vi "RT Main AB Oct 24 2019.vi"() -> ()   [LabVIEW 2018]
uses:
  Type Defs/BL Measurement States.ctl
  <vilib>/Platform/TimedLoop/XDataNode/timing_clust.ctl
  <vilib>/Platform/TimedLoop/XDataNode/nitl_modes.ctl
  <vilib>/Platform/TimedLoop/XDataNode/wakeup.ctl
  <vilib>/FPGAPlugInAG/myRIO-1900/niLvFpga_Open_myRIO-1900.vi
  <vilib>/rvi/interface/common/dynamic/niFpgaDynamicAddResources.vi
  <vilib>/Utility/error.llb/Error Cluster From Error Code.vi
  <vilib>/rvi/errors/niLvFpgaAdjustHostInterfaceError.vi
  <vilib>/FPGAPlugInAG/Dynamic/niLvFpga_Close_Dynamic.vi
  <vilib>/Platform/TimedLoop/XDataNode/XDataNode.xnode
  <vilib>/rvi/interface/nirviOpenFPGA/nirviOpenFPGA.xnode
  UNCC Watt balance Oct19/FPGA Bitfiles/UNCCWattbalanceO_FPGATarget_fpganestedFORW&R_sb-Oe1PDHtY.lvbitx
  <vilib>/rvi/interface/nirviReadWriteControl/nirviReadWriteControl.xnode
  <vilib>/rvi/interface/nirviCloseFPGA/nirviCloseFPGA.xnode
  <vilib>/Platform/TimedLoop/XDataNode/XDNodeRunTimeDep.lvlib
  NiFpgaLv.dll
  <vilib>/rvi/interface/Simulation/niFpgaSimulationCallBeginRW.vi
panel:
  out "Velocity (m/s)":dbl
  out "BL":dbl=13.526543432913298
  out "Cycles 2":dbl=2.5
  out "Time period 2":dbl=0.039999999999999994 format="%.4f"
  out "Amplitude (EMF)":dbl=0.42519521147770484 format="%.6f"
  out "Cycles":dbl=2.5
  out "Time period":dbl=0.039999999999999994 format="%.4f"
  out "Amplitude (CP)":dbl=0.00020011592768339807 format="%.6f"
  in  "no. data points":u16=500
  in  "Measure":bool
  in  "Period (us)":i64=200
  in  "EMF Gain":dbl=1.0
  in  "offset (V)":dbl format="%#_13g"
  in  "frequency (Hz)":dbl=25.0 format="%#_13g"
  in  "amplitude (V)":dbl=0.9 format="%#_13g"
  out "Late? [i-1]":bool
  in  "Stop Button":bool
  out "?":cluster{dbl, dbl}(graph)
  out "sine fit debug":dbl[][](graph)=[[-8.368204220516664e-06, -1.4715763614446807e-05, -2.4183697758518094e-05, -3.0424447258800375e-05, -3.976268367487069e-05, -4.5911881837740506e-05, -5.50670155789859e-05, -6.107125745761935e-05, -7.000514213345132e-05, -7.588731556220149e-05, -8.456180478203151e-05, -9.026850481407448e-05, -9.866071074354942e-05, -0.00010419193737888519, -0.00011230186001800507, -0.000117596579031692, -0.00012534792559927975, -0.00013041376626943556, -0.00013782179532172663, -0.00014264349909211586, -0.00014962428856981548, -0.00015414845049361426, -0.00016074014678731094, -0.00016495913758640153, -0.00017110070647115364, -0.00017500689686741834, -0.0001806754505088728, -0.0001842612112241939, -0.00018941860323176213, -0.00019267630498802198, -0.0001972843889711155, -0.0002002292903245494, -0.00020430332483940364, -0.00020683624517448153, -0.00021252768665028907, -0.00021548784655995844, -0.0002172654683613836, -0.0002196458031341074, -0.0002210572195858827, -0.00022286535849977868, -0.00022388768176755108, -0.0002251083662663838, -0.00022572633779391788, -0.00022635956787768734, -0.0002266113340555716, -0.0002266342218899247, -0.00022649689488380602, -0.000225955216137449, -0.00022539827883485657, -0.00022429966278590712, -0.00022333074446495864, -0.00022165230327906364, -0.00022029429177411228, -0.00021799787906068323, -0.0002162812914841997, -0.00021338216579947197, -0.00021127648503898553, -0.00020782042205166543, -0.00020533327738529375, -0.00020134316492973427, -0.00019848981491371278, -0.0001939198773212078, -0.00019072320978988963, -0.00018563448128538072, -0.00018208686696064813, -0.00017650223537848844, -0.00017261130353845913, -0.00016654602743488406, -0.00016234992447014657, -0.00015583452095762693, -0.00015131798831194586, -0.00014437534522483478, -0.00013962230495750486, -0.00013227531013015545, -0.00012723235729435276, -0.00011949626928300042, -0.00011423206738178433, -0.00010617554968948836, -0.00010068246944474112, -9.23284099058547e-05, -8.667511482063566e-05, -7.802351343515875e-05, -7.219474495323252e-05, -6.331426522422447e-05, -5.732528190182644e-05, -4.822355310740498e-05, -4.210487205700597e-05, -3.2835299143994996e-05, -2.6579291087477307e-05, -1.715713261211225e-05, -1.0824831774417512e-05, -1.24245845858066e-06, 5.18139371652653e-06, 1.4801913422951904e-05, 2.1256282710529914e-05, 3.0968353754367744e-05, 3.7453240154416565e-05, 4.7172940476372095e-05, 5.360442192959699e-05, 6.322494163602237e-05, 6.958775958618793e-05, 7.907858156461232e-05, 8.534221889924771e-05, 9.464993820284721e-05, 0.00010079150708759933, 0.0001098932358820208, 0.00011589747776065425, 0.00012475506965530916, 0.0001305762088591177, 0.0001391972931321238, 0.00014483532966110742, 0.00015316650136564073, 0.00015862143521979945, 0.00016660928940903606, 0.00017182771564154593, 0.00017948751087172127, 0.0001844694294825823, 0.0001917553900849901, 0.00019647028396173148, 0.00020336715138013635, 0.00020780739124464037, 0.00021426938981033606, 0.00021841208782824963, 0.00022443158826311845, 0.00022826911515632384, 0.00023377745395730651, 0.00023729455116956825, 0.00024232224544913555, 0.00024550365442421826, 0.00025001255779178165, 0.00025285827852968544, 0.0002568331324290094, 0.00025930501853914573, 0.0002623414712299921, 0.0002623414712299921, 0.0002623414712299921, 0.0002623414712299921, 0.0002623414712299921, 0.0002623414712299921, 0.0002623414712299921, 0.0002623414712299921, 0.0002623414712299921, 0.0002623414712299921, 0.0002623414712299921, 0.0002623414712299921, 0.0002623414712299921, 0.0002623414712299921, 0.0002623414712299921, 0.0002623414712299921, 0.0002623414712299921, 0.0002623414712299921, 0.0002623414712299921, 0.0002623414712299921, 0.0002623414712299921, 0.0002623414712299921, 0.0002623414712299921, 0.0002623414712299921, 0.0002623414712299921, 0.0002609605718906876, 0.00025733666478477794, 0.00025471219311228765, 0.00025048557303507935, 0.00024752541312541, 0.00024281051924866863, 0.00023946889543311405, 0.00023426572775683957, 0.00023060367426034142, 0.00022488171567206302, 0.00022090686177273901, 0.00021472714649739834, 0.0002104394921952484, 0.00020380964951096321, 0.00019926259975281132, 0.00019220551749393465, 0.0001873609258891923, 0.00017993763828066584, 0.00017486416833239232, 0.00016706704609609834, 0.0001617494392480583, 0.0001536166287745853, 0.00014808540213924953, 0.00013964742054106837, 0.00013393309123090768, 0.0001251899385080183, 0.00011929250652303274, 0.00011032047545661226, 0.00010424757007491947, 9.506954849932095e-05, 8.890509178021571e-05, 7.955159680791e-05, 7.324218380456838e-05, 6.375136182614398e-05, 5.738854387597842e-05, 4.777565344767075e-05, 4.136705982879898e-05, 3.1731281566138194e-05, 2.528454155667789e-05, 1.5664021850252515e-05, 9.270686787616142e-06, -2.964279719853011e-07, -6.651616644033151e-06, -1.609666295375132e-05, -2.2360300288386722e-05, -3.169090742633932e-05, -3.783247631109144e-05, -4.700286860857226e-05, -5.303762759967652e-05, -6.201728794421471e-05, -6.792997848543571e-05, -7.666550193020736e-05, -8.240271907472114e-05, -9.091699345407936e-05, -9.645584936753283e-05, -0.00010466495262218286, -0.00011001307658269371, -0.00011787886232204706, -0.0001230515128858507, -0.00013056635183178965, -0.0001354490898271205, -0.00014262061125776276, -0.00014724395379709168, -0.00015398823565314246, -0.00015834455345835173, -0.00016463870790545793, -0.0001686669667516059, -0.00017452625234600297, -0.00017823408151120733, -0.00018360509330607133, -0.00018700775134656753, -0.0001918599722294276, -0.00019491168347650942, -0.00019923748416924783, -0.00020194587790103294, -0.00020572999984741437, -0.00020807981750766737, -0.00021127648503898553, -0.0002132295802371179, -0.00021589982757831447, -0.00021748671742679703, -0.00021958476890916577, -0.00022076730701740992, -0.00022227027480659772, -0.0002230866075651921, -0.00022404026732990518, -0.0002244446190701435, -0.00022481082441979332, -0.00022483371225414644, -0.0002246048339106153, -0.0002242691456734363, -0.00022343755435860651, -0.00022269751438118917, -0.0002212632100950607, -0.00022013407693364048, -0.0002181352060668019, -0.00021660935044326098, -0.00021402302516135917, -0.00021210044707569762, -0.0002089571844912034, -0.00020664551322153893, -0.00020293005477821683, -0.00020024454888078482, -0.00019598741169110575, -0.00019295858827837704, -0.000184749485023727, -0.00017945476601004007, -0.00017572404901048256, -0.00016991816836290944, -0.00016588228023864377, -0.00015958812579153756, -0.0001552623250987991, -0.00014853330179898374, -0.00014390232998153708, -0.0001367842134977188, -0.00013189384622427021, -0.00012435611944397817, -0.00011922924454888077, -0.00011137871736576284, -0.00010600770557089886, -9.782911942871964e-05, -9.227500495903076e-05, -8.381413552649647e-05, -7.809217693821809e-05, -6.937191204968184e-05, -6.349736789904938e-05, -5.456348322321741e-05, -4.852109495399546e-05, -3.938884904710317e-05, -3.3232021606115636e-05, -2.392430230251614e-05, -1.766829424599845e-05, -8.223247936280279e-06, -1.8985763767032463e-06, 7.668538382898196e-06, 1.404661488929916e-05, 2.3659505317606828e-05, 3.009861604894943e-05, 3.9742023589727915e-05, 4.6173505042952805e-05, 5.578639547126048e-05, 6.213395486519063e-05, 7.164003539985044e-05, 7.790367273448582e-05, 8.726479698490926e-05, 9.343688298213219e-05, 0.00010259201672337759, 0.00010864966354883496, 0.00011757591894654922, 0.0001234580923752994, 0.00013219361582007106, 0.00013789268657399633, 0.0001463459267284129, 0.00015187715336374867, 0.00016001759311533938, 0.000165319941407144, 0.00017312469292155572, 0.00017822867998230002, 0.0001856672261470619, 0.0001905423348642751, 0.0001975689000106809, 0.00020214646688130364, 0.00020879156812182424, 0.00021307922242397417, 0.00021925130842119712, 0.00022323379159863886, 0.00022897100874315265, 0.00023264069151776853, 0.0002378972641408669, 0.0002412236294001861, 0.00024597666966751596, 0.00024895208813342074, 0.0002531863374887467, 0.0002558184384393548, 0.00025951863832644143, 0.0002617997924836351, 0.0002623414712299921, 0.0002623414712299921, 0.0002623414712299921, 0.0002623414712299921, 0.0002623414712299921, 0.0002623414712299921, 0.0002623414712299921, 0.0002623414712299921, 0.0002623414712299921, 0.0002623414712299921, 0.0002623414712299921, 0.0002623414712299921, 0.0002623414712299921, 0.0002623414712299921, 0.0002623414712299921, 0.0002623414712299921, 0.0002623414712299921, 0.0002623414712299921, 0.0002623414712299921, 0.0002623414712299921, 0.0002623414712299921, 0.0002623414712299921, 0.0002623414712299921, 0.0002623414712299921, 0.0002596407067763247, 0.00025720696705677695, 0.0002532931473823946, 0.000250493202313197, 0.0002460605917268107, 0.00024288681202984567, 0.00023792778125333774, 0.00023444883043166446, 0.00022897100874315265, 0.0002251716282405358, 0.00021924367914307944, 0.00021512386895951898, 0.0002087305338968826, 0.00020432844042296712, 0.00019750786578573928, 0.00019282348902146873, 0.00018559856264400258, 0.00018067004897996545, 0.0001678528617422219, 0.0001599107832216915, 0.00015450925431435673, 0.00014624674611288274, 0.00014061633886201683, 0.00013206391809207009, 0.00012625803744449696, 0.00011743096266231285, 0.00011144960861803251, 0.00010237076765796416, 9.629023299815366e-05, 8.702828936326041e-05, 8.081042769733124e-05, 7.1418786334437e-05, 6.509411477485997e-05, 5.559566351831787e-05, 4.9217587011916905e-05, 3.962758441796235e-05, 3.322662007720827e-05, 2.3628988205136012e-05, 1.722802386438194e-05, 7.668538382898196e-06, 1.3057204327326442e-06, 0.0], [0.01724705128400751, 0.030827166333521522, 0.04379693913361917, 0.0648537467384836, 0.07721317728916488, 0.09750705708225885, 0.11047682988235649, 0.1304655385507423, 0.14343531135083995, 0.16296626333216346, 0.17547827944519884, 0.19485664586416826, 0.20706349085249548, 0.22598410058440263, 0.23742801776095937, 0.2560434563681584, 0.26870805804354786, 0.2861028121519141, 0.29724155820376263, 0.31387338450035845, 0.3254698872392693, 0.34133878572409465, 0.3523249462135892, 0.3678886735737063, 0.377501564002014, 0.3929127057997771, 0.40252559622808476, 0.41610571127759877, 0.4258711872682605, 0.43823061781894185, 0.4458598959366463, 0.45776156980026533, 0.46584860460503213, 0.4765295939698184, 0.48339594427575244, 0.4936191769534765, 0.5003329416970564, 0.5088777331888855, 0.5143708134336328, 0.5221526771136913, 0.5265776584219599, 0.533444008727894, 0.5364957199749758, 0.5421413857820772, 0.5448879259044508, 0.5485499794009489, 0.550533591711552, 0.5531275462715716, 0.5549585730198207, 0.5557215008315911, 0.5558740863939452, 0.5563318430810075, 0.5554163297068829, 0.5541956452080502, 0.5523646184598011, 0.5503810061491979, 0.5482448082762407, 0.5438198269679722, 0.5413784579703067, 0.5357327921632054, 0.5311552252925826, 0.5239837038619404, 0.5191009658666096, 0.5110139310618428, 0.5053682652547414, 0.4957553748264337, 0.48843126783343743, 0.4786657918427757, 0.47103651372507116, 0.4595925965485144, 0.4508952194943313, 0.43853578894365, 0.43029616857652914, 0.41641088240230695, 0.40740833422341566, 0.3926075346750689, 0.3829946442467612, 0.3671257457619359, 0.3576654408959823, 0.34149137128644874, 0.3314207241710788, 0.31417855562506664, 0.3030398095732181, 0.2857976410272059, 0.274048552725941, 0.25772189755405334, 0.2462779803774966, 0.22766254177029763, 0.2172867235302195, 0.19851869936066643, 0.18722736774646376, 0.1686119291392648, 0.1564050841509376, 0.13763705998138454, 0.12619314280482777, 0.10635701969879607, 0.09369241802340661, 0.07553473610326988, 0.06348047667729678, 0.04410211025832735, 0.03159009414529197, 0.012822069975738903, 0.000615224987411702, -0.01830538474449546, -0.030207058608114477, -0.04989059615179208, -0.06225002670247338, -0.08117063643438055, -0.09307231029799956, -0.1121455055922608, -0.12374200833117166, -0.14251003250072472, -0.1538013641149274, -0.17287455940918864, -0.18431847658574538, -0.2011028884446953, -0.21392007568243884, -0.23039931641668057, -0.2426061614050078, -0.25954315882631174, -0.27068190487816035, -0.28655080336298566, -0.2969266216030638, -0.3129481056502433, -0.3233239238903214, -0.3384298945633763, -0.3489582983658085, -0.3625384134153225, -0.37230388940598425, -0.38527366220608195, -0.39381845369791096, -0.40739856874742497, -0.41472267574042126, -0.42662434960404033, -0.4344062132840989, -0.4449346170865311, -0.45225872407952744, -0.46126127225841873, -0.46766986587729054, -0.4756043151197032, -0.4807922242397422, -0.48842150235744675, -0.492236141416299, -0.498949906159879, -0.502306788531669, -0.5073421120893539, -0.5096308955246652, -0.5131403634588093, -0.5151239757694125, -0.5174127592047238, -0.5181756870164943, -0.5197015426400352, -0.5195489570776811, -0.5192437859529729, -0.5184808581412025, -0.516039489143537, -0.5148188046447043, -0.5119196789599766, -0.5088679677128948, -0.5036800585928558, -0.5009335184704822, -0.4952878526633808, -0.49147321360452856, -0.4841491066115322, -0.4788086119291391, -0.4710267482490805, -0.4653810824419792, -0.45531043532660925, -0.44890184170773745, -0.43822085234295116, -0.4310493309123089, -0.41960541373575216, -0.41090803668156906, -0.3985486061308878, -0.3900038146390587, -0.37581335734012833, -0.36665822359888295, -0.35139966736347394, -0.3417867769351663, -0.3265282206997573, -0.3153894746479087, -0.2992154050383752, -0.2889921723606511, -0.271902589376993, -0.2604586722004363, -0.24306391809207006, -0.2313148297908051, -0.21254680562125203, -0.20018737507057074, -0.1826400353998504, -0.16982284816210683, -0.15074965286784558, -0.13747470894303976, -0.11794375696171625, -0.10558432641103493, -0.08513786105558688, -0.0727784305049056, -0.0527897218365198, -0.03920960678700579, -0.019220898118619996, -0.0060985397561682565, 0.014195340036925713, 0.027165112837023362, 0.04745899263011733, 0.060428765430214984, 0.08026488853624669, 0.09399758914811479, 0.11307078444237603, 0.12604055724247368, 0.14618185147321355, 0.1589990387109571, 0.17837740512992656, 0.19073683568060784, 0.20981003097486908, 0.22247463265025855, 0.24093748569510345, 0.25207623174695204, 0.2703864992294428, 0.2827459297801241, 0.2990725849520117, 0.31066908769092255, 0.32745349954987246, 0.338439660039367, 0.3540033873994841, 0.36453179120191637, 0.3794851763126172, 0.3895558234279871, 0.41320658559287105, 0.42678670064238505, 0.43502632100950595, 0.4476909226848954, 0.45562537192730806, 0.4666115324168026, 0.47317271159802843, 0.484311457649877, 0.49010970901933243, 0.4994174283229319, 0.5050630941300333, 0.5134553000595082, 0.5191009658666096, 0.5258147306101895, 0.5297819552313958, 0.5357327921632054, 0.5390896745349953, 0.5432094847185558, 0.5458034392785752, 0.5496180783374275, 0.5506861772739061, 0.5528223751468634, 0.5535853029586338, 0.5541956452080502, 0.5540430596456961, 0.5535853029586338, 0.5528223751468634, 0.5506861772739061, 0.5483973938385948, 0.5464137815279916, 0.5430568991562017, 0.538479332285579, 0.5348172787890808, 0.5290190274196254, 0.5239837038619404, 0.5174225246807146, 0.5117768588736132, 0.5030794818194301, 0.4975864015746828, 0.4873631688969588, 0.48171750308985745, 0.4699684147885925, 0.4617287944214717, 0.45028487724491495, 0.44189267131543997, 0.42861772739063414, 0.41992035033645103, 0.40588247859987475, 0.39626958817156704, 0.3811636174985122, 0.3713981415078504, 0.3562921708347955, 0.3451534247829469, 0.3286741840487052, 0.318145780246273, 0.3007510261379067, 0.28945969452370407, 0.27267528266475416, 0.26062102323878106, 0.24414178250453933, 0.23178235195385805, 0.2143875978454918, 0.2020281672948105, 0.18448082762409015, 0.17090071257457615, 0.15350595846620987, 0.14190945572729904, 0.12268367487068371, 0.11062941544471058, 0.09170880571280343, 0.0801123029738926, 0.060733936554923165, 0.04745899263011733, 0.028843554022918355, 0.016789294596945243, -0.0016735584478996465, -0.01479591681035139, -0.033411355417550366, -0.04546561484352348, -0.06484398126249291, -0.07674565512611192, -0.09597143598272728, -0.10802569540870038, -0.12572562064177484, -0.1368643666936234, -0.15517463417611418, -0.16783923585150368, -0.1856917466469322, -0.1975934205105512, -0.2148355890565634, -0.2268898484825365, -0.24321650365442415, -0.2549655919556891, -0.271750003814639, -0.2822784076170712, -0.29784213497718837, -0.3080653676549124, -0.32408685170209184, -0.3336997421303995, -0.3485005416787462, -0.3579608465446998, -0.37215130384363015, -0.38176419427193786, -0.39427621038497324, -0.40236324518974, -0.41487526130277536, -0.42280971054518807, -0.43379587103468253, -0.44142514915238706, -0.4508854540183406, -0.45775180432427465, -0.46736469475258235, -0.47285777499732956, -0.4844542777362404, -0.49147321360452856, -0.495593023788089, -0.5013912751575444, -0.503985229717564, -0.5082576254634784, -0.5106989944611439, -0.5135981201458716, -0.5146662190823502, -0.516039489143537, -0.5168024169553075, -0.5166498313929534, -0.5169550025176616, -0.5149713902070584, -0.5139032912705798, -0.5103938233364357, -0.5096308955246652, -0.5053584997787508, -0.502306788531669, -0.497271464973984, -0.49345682591513174, -0.48659047560919766, -0.48170773761386676, -0.47453621618322456, -0.46889055037612326, -0.4598880021972319, -0.45393716526542244, -0.44371393258769837, -0.43684758228176435, -0.4250984939804994, -0.41807955811221126, -0.40572012756153, -0.39702275050734687, -0.3840529777072492, -0.3747452584036497, -0.36024962998001114, -0.35124708180111985, -0.3364462822527731, -0.3259178784503409, -0.31004897996551556, -0.29952057616308336, -0.2833465065535498, -0.2715974182522849, -0.25527076308039726, -0.24306391809207006, -0.2253639928589956, -0.21376749012008475, -0.19545722263759396, -0.18370813433632902, -0.16524528129148414, -0.1521229229290324, -0.13320231319712525, -0.12084288264644394, -0.10131193066512043, -0.08834215786502278, -0.06804827807192879, -0.0558414330836016, -0.03570013885286172, -0.022730366052764066, -0.0030468285090864584]]
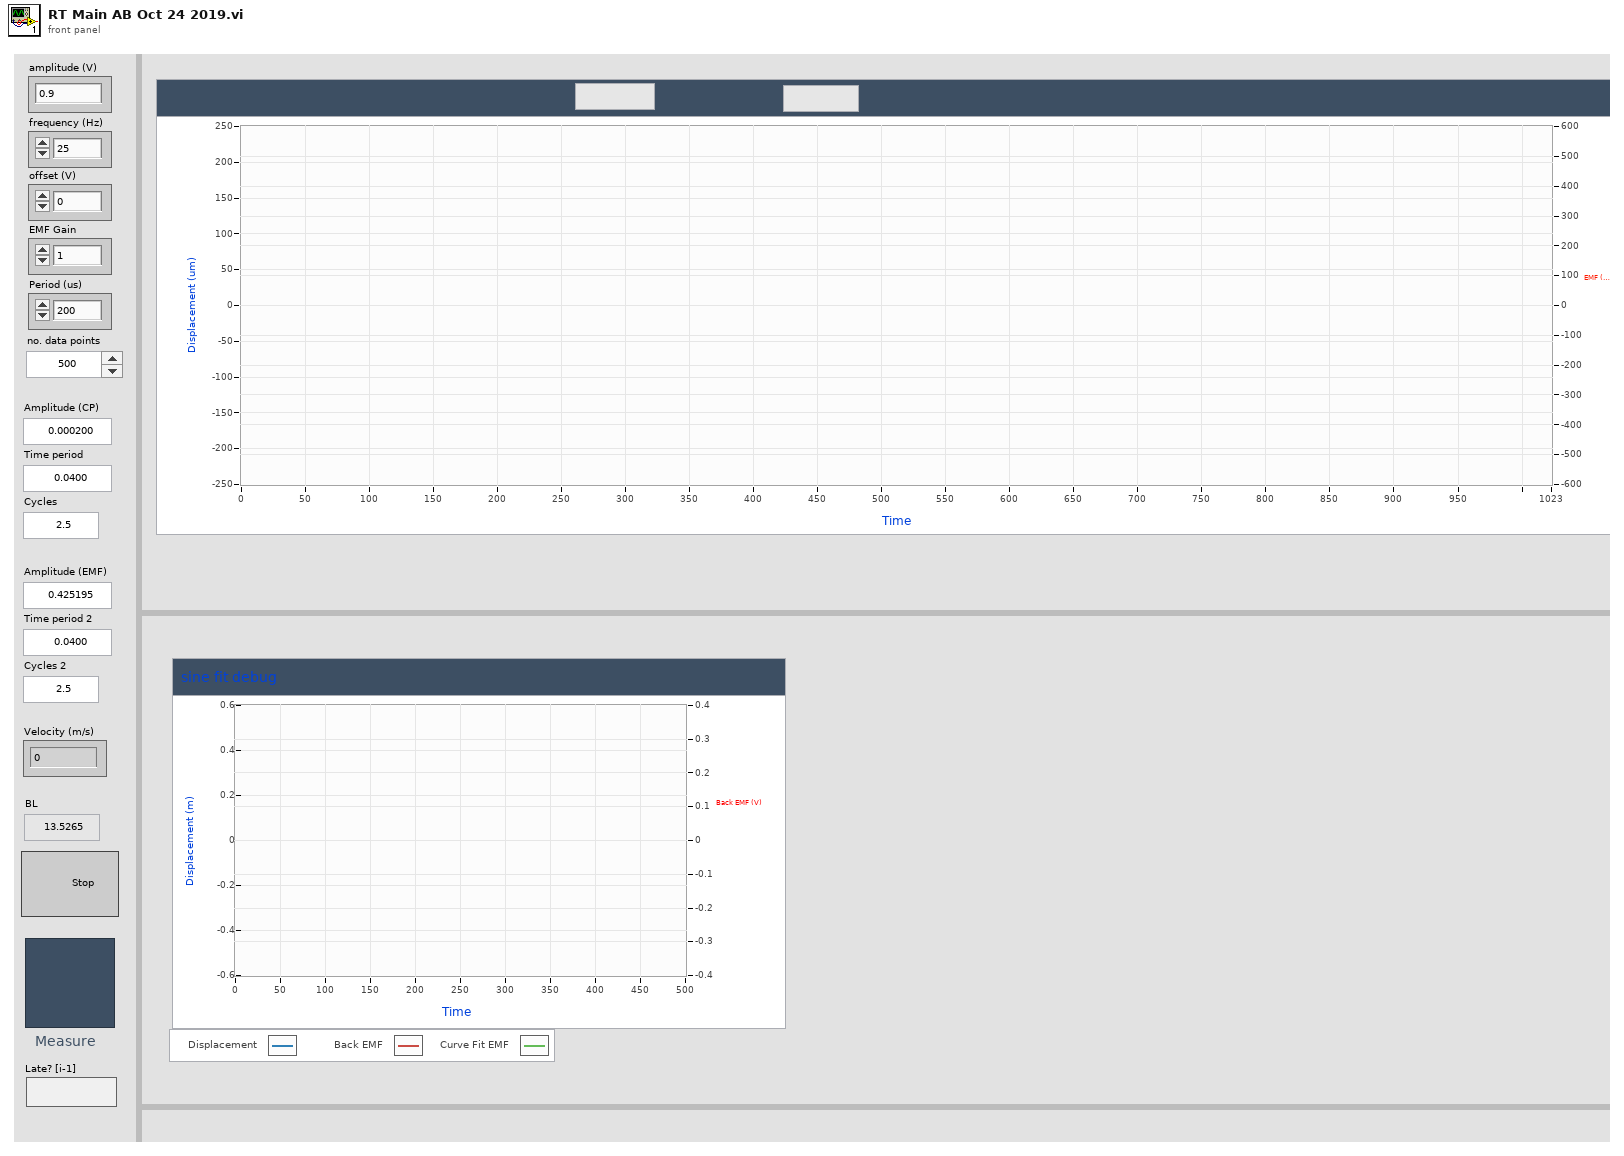
[diagram p1: front panel]
types:
  T1 = typedef "BL Measurement States.ctl" = enum16{"idle", "initialize", "collect data", "prepare data", "fit sine", "calculate BL", "exit meas"}
  T2 = typedef "XDNodeRunTimeDep.lvlib/timing_clust.ctl" = cluster{"Expected End [f-1]":u64, "Actual End [f-1]":u64, "Finished Late? [f-1]":bool, "Expected End [i-1]":u64, "Actual End [i-1]":u64, "Finished Late? [i-1]":bool, "Expected Start [i]":u64, "Actual Start [i]":u64, "Expected Start [f]":u64, "Actual Start [f]":u64, "Source Name":string, "Structure Name":string, "Period":i64, "Deadline":i64, "Offset":i64, "Start":i64, "Priority":i32, "Timeout":i32, "Mode":T3, "Wakeup Reason":T4, "Error":errorcluster, "Source Type":string, "Secondary Source Type":string, "Global End Time":u64, "Global Start Time":u64, "Frame Duration":u64, "Iteration Duration":u64, "Assigned CPU":i32, "I/O Scan Engine Mode":u32}
  T3 = typedef "XDNodeRunTimeDep.lvlib/nitl_modes.ctl" = enum32{"No Change", "Process missed periods, maintain original phase", "Discard missed periods, maintain original phase", "Process missed periods, ignore original phase", "Discard missed periods, ignore original phase"}
  T4 = typedef "XDNodeRunTimeDep.lvlib/wakeup.ctl" = enum32{"Normal", "Aborted", "Asynchronous wakeup", "Timing source error", "Timed loop error", "Timeout"}
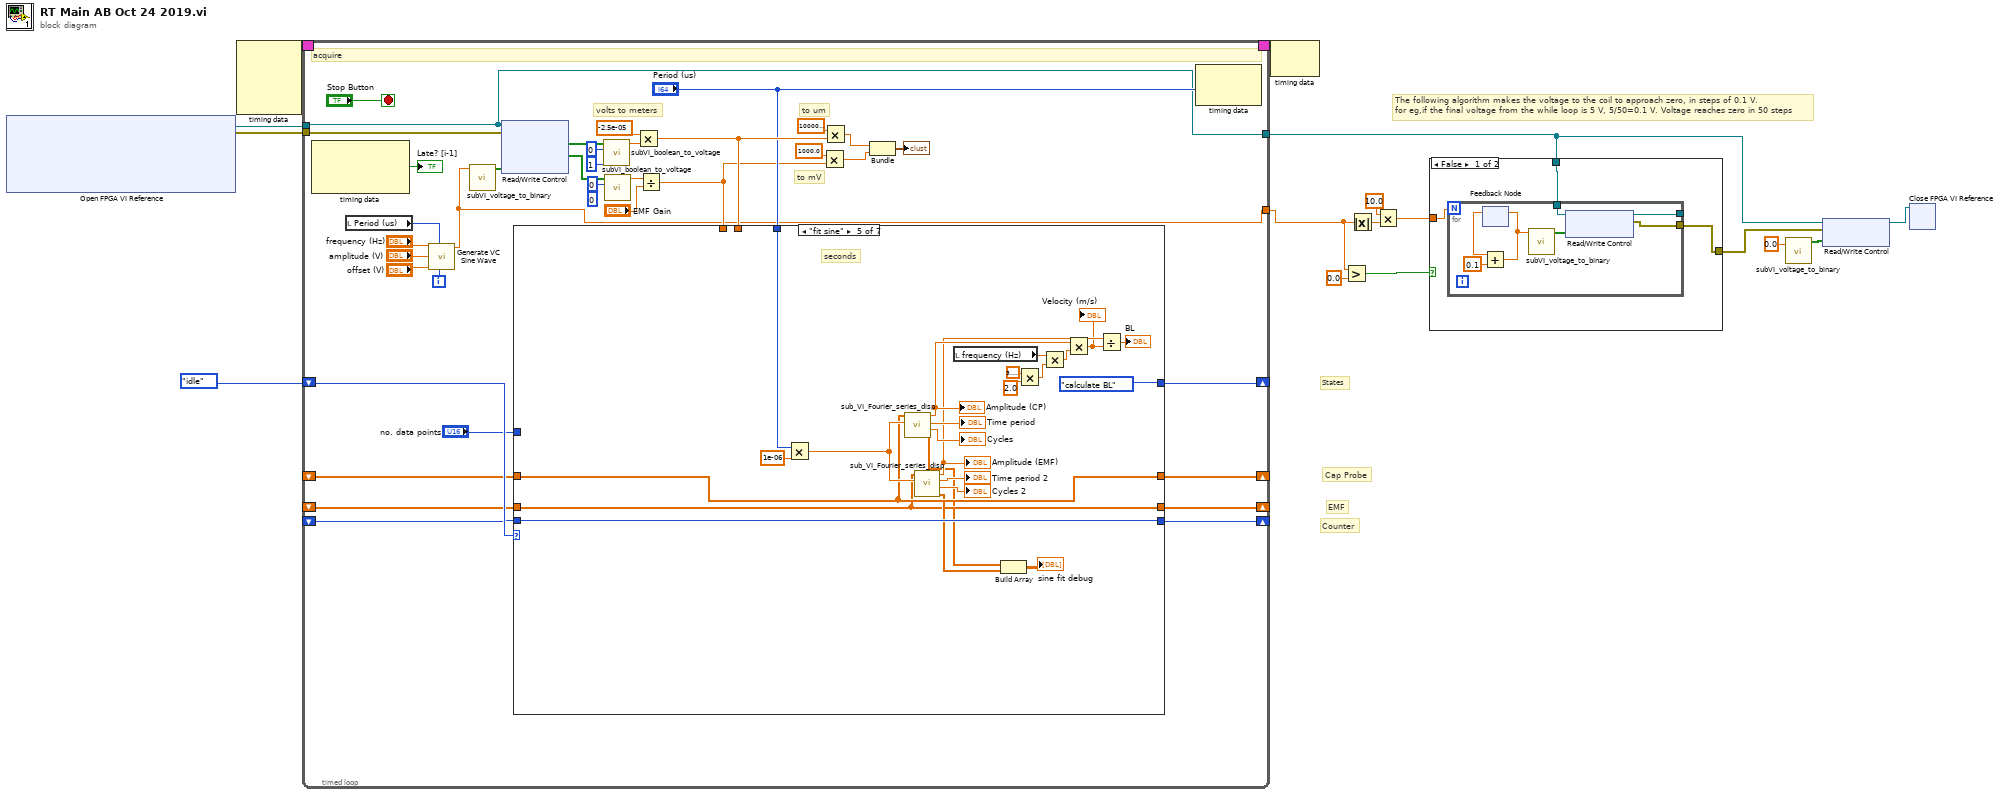
[diagram p0: block diagram]
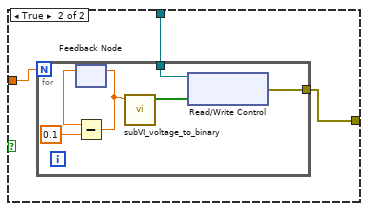
[diagram p2: hidden frame]
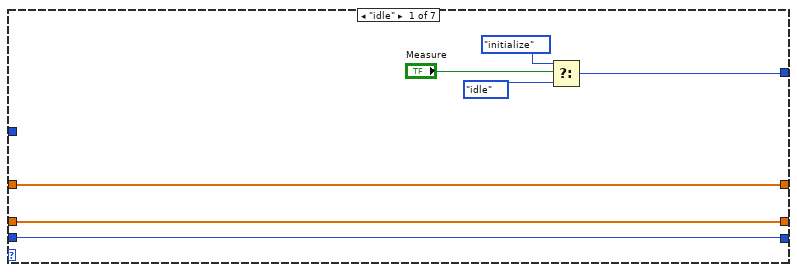
[diagram p3: hidden frame]
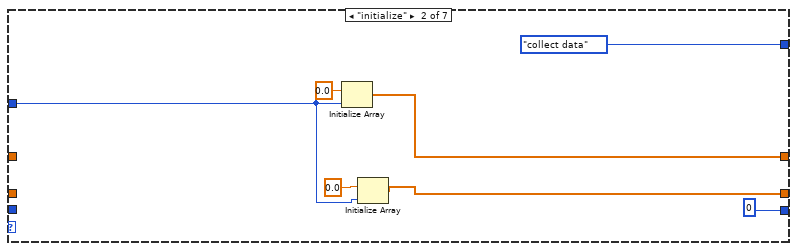
[diagram p4: hidden frame]
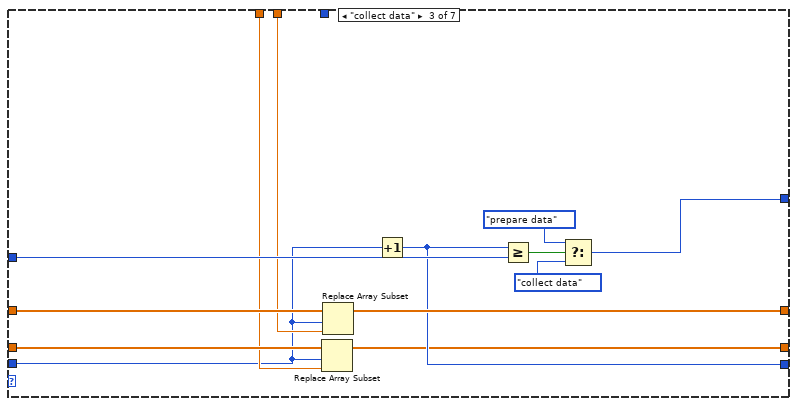
[diagram p5: hidden frame]
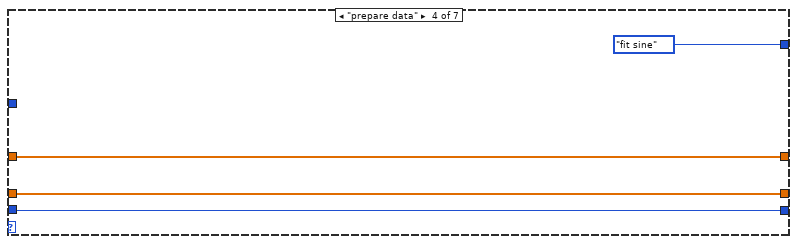
[diagram p6: hidden frame]
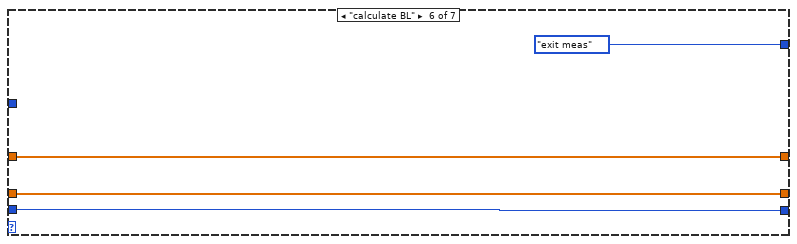
[diagram p7: hidden frame]
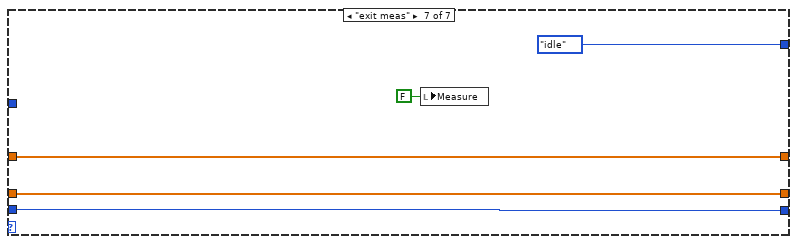
[diagram p8: hidden frame]
diagram:
  # "The following algorithm makes the voltage to the coil to approach zero, in steps of 0.1 V.\nfor eg,if the final voltage from the while loop is 5 V, 5/50=0.1 V. Voltage reaches zero in 50 steps"
  # "States"
  # "Counter"
  # "EMF"
  # "Cap Probe"
  n1 = xnode "Open FPGA VI Reference"() -> ("FPGA VI Reference Out"=w14:refnum<k20>, "error out"=w13:errorcluster)  [unwired: 2 in]
  n2 = node-c288() -> (w16:T2)  [unwired: 4 in]
  n3 = timed-loop {
    timing: w16 -> [_]
    timing-out: [_] -> w15
    tunnel: w14 -> [w17]
    tunnel: w13 -> [w44]
    shift-right: [w37] -> _
    shift-left: BL_Measurement_States."idle" ("BL meas states") -> [w38]
    shift-right: [w36] -> _
    shift-left: _ -> [w35]
    shift-right: [w33] -> _
    shift-left: _ -> [w34]
    shift-right: [w25] -> _
    shift-left: _ -> [w26]
    tunnel: [w18] -> w2
    tunnel: [w17] -> w1
    i -> [w53]
    stop <- "Stop Button" stop-if-true
    (unwired) i16 0 ("Gain")
    # "to mV"
    # "to um"
    # "volts to meters"
    # "acquire"
    n4 = node-c288() -> (→"Late? [i-1]":bool)  [unwired: 1 in, 2 out]
    n5 = local read "Period (us)"() -> (w48:i64)
    n6 = call "Generate VC Sine Wave.vi"("Counter"=w53, "Period (us)"=w48, "offset (V)"="offset (V)", "amplitude (V)"="amplitude (V)", "frequency (kHz)"="frequency (Hz)") -> ("V"=w18:dbl)  [unwired: 6 in]
    n7 = call "subVI_voltage_to_binary.vi"("voltage"=w18) -> ("binary"=w45:bool[])  [unwired: 10 in]
    n8 = xnode "Read/Write Control"("FPGA VI Reference In"=w17, "error in"=w44, "DAC 1 write"=w45) -> ("ADC  1 R"=w40:bool[], "ADC 2 R"=w39:bool[])  [unwired: 2 out]
    n9 = call "subVI_boolean_to_voltage.vi"("Gain"=i16 1, "UNI"=i16 0, "ADC read"=w40) -> ("V"=w32:dbl)  [unwired: 8 in]
    n10 = call "subVI_boolean_to_voltage.vi"("UNI"=i16 0, "ADC read"=w39) -> ("V"=w31:dbl)  [unwired: 9 in]
    n11 = Multiply(x=-2.5e-05, y=w32) -> (x*y=w30:dbl)
    n12 = Divide(x=w31, y="EMF Gain") -> (x/y=w27:dbl)
    n13 = case shown="\"fit sine\"" w38 {
      tunnel: [w58 BL_Measurement_States."collect data" ("BL meas states") w74 BL_Measurement_States."fit sine" ("BL meas states") BL_Measurement_States."calculate BL" ("BL meas states") BL_Measurement_States."exit meas" ("BL meas states") BL_Measurement_States."idle" ("BL meas states")] -> w37
      tunnel: [w55 w63 w75 w82 w90 w110 w115] -> w36
      tunnel: [w54 w62 w70 w81 w87 w108 w112] -> w25
      tunnel: w35 -> [w55 _ w77 w82 w90 w110 w115]
      tunnel: w34 -> [w56 _ w68 w84 w107 w109 w114]
      tunnel: [w56 0 w72 w84 w107 w109 w114] -> w33
      tunnel: "no. data points" -> [_ w61 w76 _ _ _ _]
      tunnel: w30 -> [_ _ w73 _ _ _ _]
      tunnel: "Period (us)" -> [_ _ _ _ w104 _ _]
      tunnel: w27 -> [_ _ w69 _ _ _ _]
      tunnel: w26 -> [w54 _ w71 w81 w87 w108 w112]
      frame "idle" {
        n14 = Select(t=BL_Measurement_States."initialize" ("BL meas states"), s="Measure", f=BL_Measurement_States."idle" ("BL meas states 2")) -> (s? t:f=w58:T1)
      }
      frame "initialize" {
        n15 = Initialize Array(0.0 ("element"), w61) -> (w63:dbl[])
        n16 = Initialize Array(0.0 ("element"), w61) -> (w62:dbl[])
      }
      frame "collect data" {
        n17 = Replace Array Subset(array=w71, new element=w69, index=w68) -> (w70:dbl[])
        n18 = Replace Array Subset(array=w77, new element=w73, index=w68) -> (w75:dbl[])
        n19 = Increment(x=w68) -> (x+1=w72:i32)
        n20 = Greater Or Equal?(x=w72, y=w76) -> (x >= y?=w78:bool)
        n21 = Select(t=BL_Measurement_States."prepare data" ("BL meas states"), s=w78, f=BL_Measurement_States."collect data" ("BL meas states 2")) -> (s? t:f=w74:T1)
      }
      frame "prepare data" {
      }
      frame "fit sine" {
        # "seconds"
        n22 = Multiply(x=w104, y=1e-06) -> (x*y=w92:dbl)
        n23 = call "sub_VI_Fourier_series_disp.vi"("del t"=w92, "x,i"=w90) -> ("clipped array"=w85:dbl[], "number of cycles"=→"Cycles":dbl, "Time period"=→"Time period":dbl, "computed amplitude"=w99:dbl)  [unwired: 6 in]
        "Amplitude (CP)" <- w99
        n24 = call "sub_VI_Fourier_series_disp.vi"("del t"=w92, "x,i"=w87) -> ("clipped array"=w88:dbl[], "number of cycles"=→"Cycles 2":dbl, "Time period"=→"Time period 2":dbl, "computed amplitude"=w91:dbl)  [unwired: 6 in]
        "Amplitude (EMF)" <- w91
        n25 = local read "frequency (Hz)"() -> (w93:dbl)
        n26 = Build Array(w85, w88) -> (→"sine fit debug":dbl[][])
        n27 = Multiply(x=3.141592653589793, y=2.0) -> (x*y=w97:dbl)
        n28 = Multiply(x=w93, y=w97) -> (x*y=w94:dbl)
        n29 = Multiply(x=w99, y=w94) -> (x*y=w86:dbl)
        "Velocity (m/s)" <- w86
        n30 = Divide(x=w91, y=w86) -> (x/y=→"BL":dbl)
      }
      frame "calculate BL" {
      }
      frame "exit meas" {
        n31 = local write "Measure"(FALSE) -> ()
      }
    }
    n32 = Multiply(x=1000.0, y=w27) -> (x*y=w21:dbl)
    n33 = Multiply(x=1000000.0, y=w30) -> (x*y=w19:dbl)
    n34 = Bundle(w19, w21) -> (→"?":cluster{dbl, dbl})  [unwired: 1 in]
    n35 = node-c288("Period (us)") -> ()  [unwired: 1 in, 1 out]
  }
  n36 = node-c288(w15) -> ()  [unwired: 1 out]
  n37 = Greater?(x=w2, y=0.0) -> (0:w11:bool)
  n38 = Absolute Value(x=w2) -> (abs(x)=w7:dbl)
  n39 = Multiply(x=10.0, y=w7) -> (x*y=w10:dbl)
  n40 = case shown="False" w11 {
    tunnel: w10 -> [w124 w134]
    tunnel: w1 -> [w123 w133]
    tunnel: [w122 w132] -> w3
    frame False {
      n41 = for {
        N: w124 -> [_]
        tunnel: [w130] -> _
        tunnel: [w126] -> w122
        tunnel: w123 -> [w125]
        n42 = feedback #1() -> (w128:dbl)  [unwired: 1 in]
        n43 = Add(x=w128, y=0.1) -> (x+y=w127:dbl)
        n44 = feedback-in #1(w127) -> ()
        n45 = call "subVI_voltage_to_binary.vi"("voltage"=w127) -> ("binary"=w131:bool[])  [unwired: 10 in]
        n46 = xnode "Read/Write Control"("FPGA VI Reference In"=w125, "DAC 1 write"=w131) -> ("FPGA VI Reference Out"=w130:refnum<k20>, "error out"=w126:errorcluster)  [unwired: 1 in]
      }
    }
    frame True {
      n47 = for {
        N: w134 -> [_]
        tunnel: [w136] -> w132
        tunnel: w133 -> [w135]
        n48 = feedback #2() -> (w139:dbl)  [unwired: 1 in]
        n49 = Subtract(x=w139, y=0.1) -> (x-y=w137:dbl)
        n50 = feedback-in #2(w137) -> ()
        n51 = call "subVI_voltage_to_binary.vi"("voltage"=w137) -> ("binary"=w140:bool[])  [unwired: 10 in]
        n52 = xnode "Read/Write Control"("FPGA VI Reference In"=w135, "DAC 2 write"=w140) -> ("error out"=w136:errorcluster)  [unwired: 1 in, 1 out]
      }
    }
  }
  n53 = call "subVI_voltage_to_binary.vi"("voltage"=0.0) -> ("binary"=w5:bool[])  [unwired: 10 in]
  n54 = xnode "Read/Write Control"("FPGA VI Reference In"=w1, "error in"=w3, "DAC 1 write"=w5) -> ("FPGA VI Reference Out"=w6:refnum<k20>)  [unwired: 1 out]
  n55 = xnode "Close FPGA VI Reference"("FPGA VI Reference In"=w6) -> ()  [unwired: 1 in, 1 out]
